vi "_Dequeue CSMQ.vi"(8 "Error in":errorcluster caption="Error in (no error)", 9 "Dequeue Timeout(0ms)":i32, 10 "State(s) in (\"\")":string, 11 "CSMQ in":T1) -> (0 "Error out":errorcluster, 2 "States Out":string, 3 "CSMQ out":T1)   [LabVIEW 2014, in "Communicable State Machine.lvlib"]
uses:
  Communicable State Machine.lvlib
  _CSMObj.ctl
  Priority Queue/Priority Queue.lvclass
  Typedef/_CSM_MODE.ctl
  _CSMObj-Data.ctl
  Typedef/_CSM Status Change Event Data.ctl
  Priority Queue/Priority Queue.lvclass/Priority Queue.ctl
  AdvanceAPI/CSM - Message Type.ctl
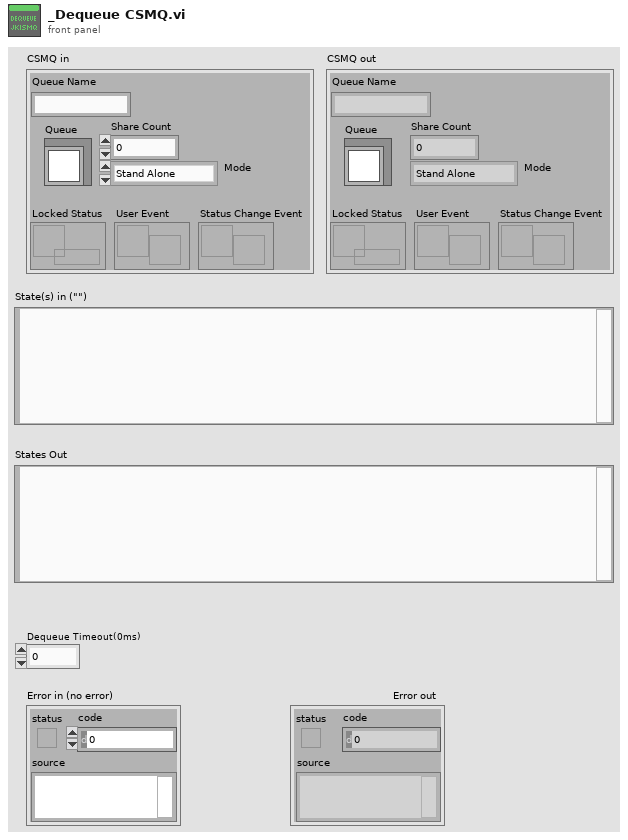
[diagram p1: front panel]
types:
  T1 = typedef "Communicable State Machine.lvlib/_CSMObj.ctl" = cluster{"Queue Name":string, "Mode":T2, "Share Count":i32, "Queue":refnum<class "Priority Queue.lvclass">, "Locked Status":refnum<data-value>, "User Event":refnum<user-event>, "Status Change Event":refnum<user-event>}
  T2 = typedef "Communicable State Machine.lvlib/_CSM_MODE.ctl" = enum16{"Stand Alone", "CSM", "Action Worker"}
  T3 = typedef "Communicable State Machine.lvlib/CSM - Message Type.ctl" = enum16{"Async", "Async without Reply", "Sync"}
  T4 = typedef "_CSMObj-Data.ctl" = cluster{"Locked?":bool, "RemoteMessge?":bool}
  T5 = typedef "Communicable State Machine.lvlib/_Cross CSM State Data.ctl" = cluster{"Msg Type":T6, "state":string, "args":string, "source":string, "RespQ":refnum<queue>, "Response For Message":T7, "Target":string}
  T6 = typedef "Communicable State Machine.lvlib/_CSM_MSG_TYPE.ctl" = enum16{"Sync Message(-@)", "Async Message(->)", "Async without Response(->|)", "Async Response", "Broadcast(-><status>)", "Broadcast(-><interrupt>)", "Request to Post Message", "Request to Post Message without Reply", "Request to Publish Status"}
  T7 = typedef "Communicable State Machine.lvlib/_CSM_Response Source Message.ctl" = cluster{"State":string, "Arguments":string, "Error":errorcluster}
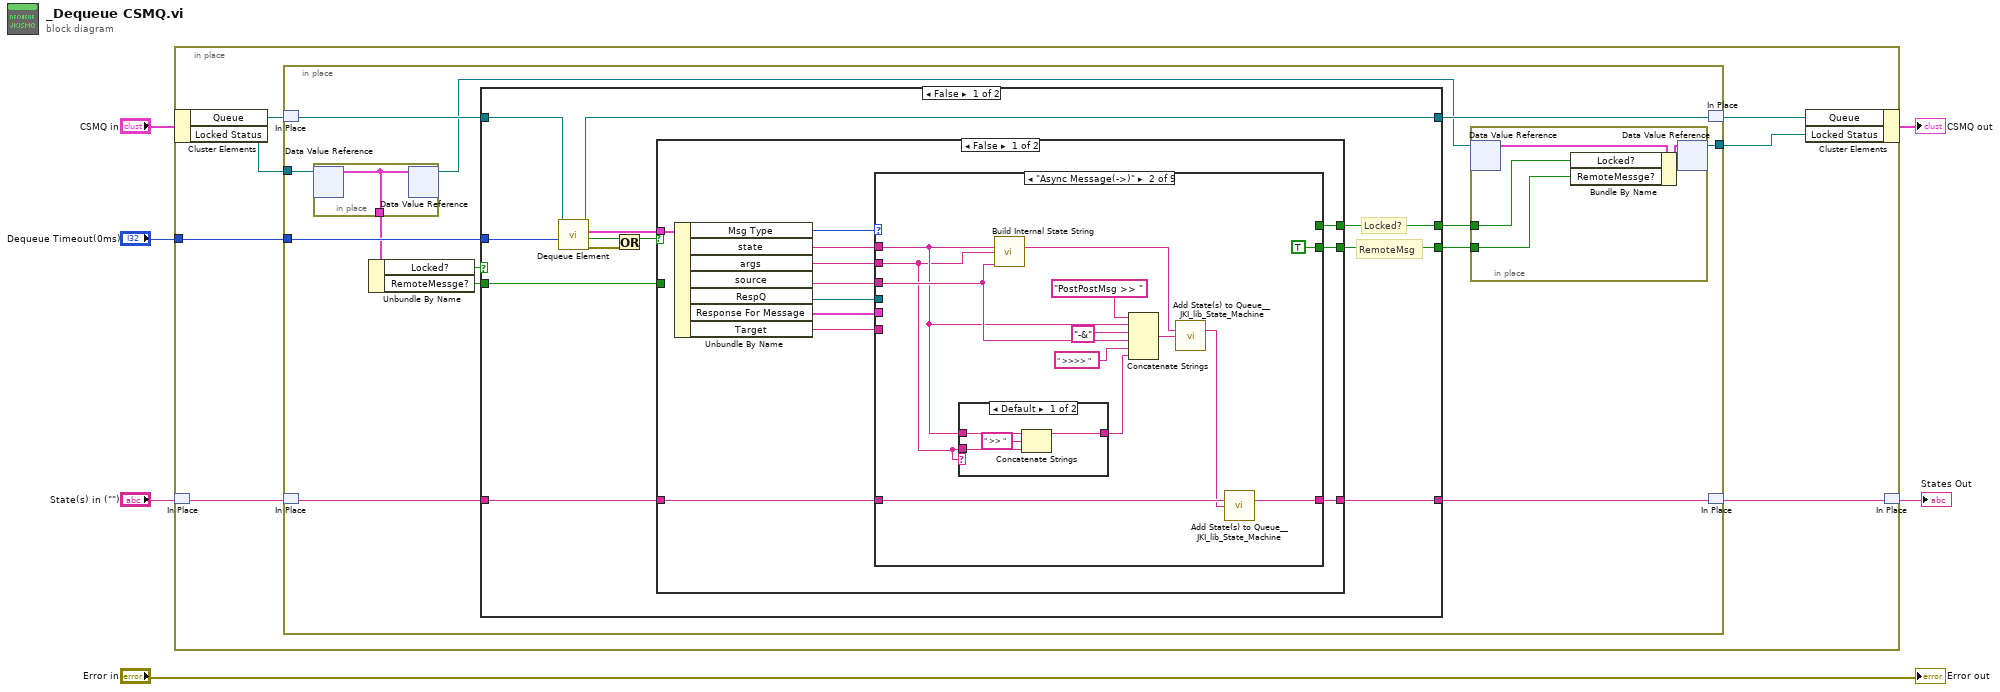
[diagram p0: block diagram]
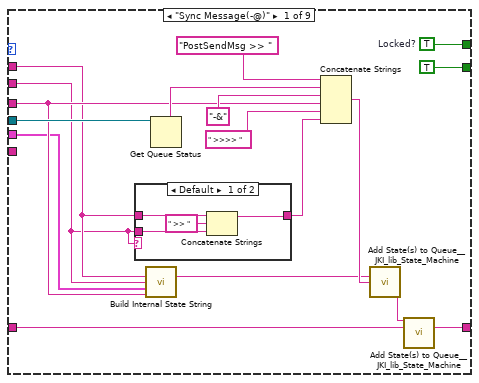
[diagram p2: hidden frame]
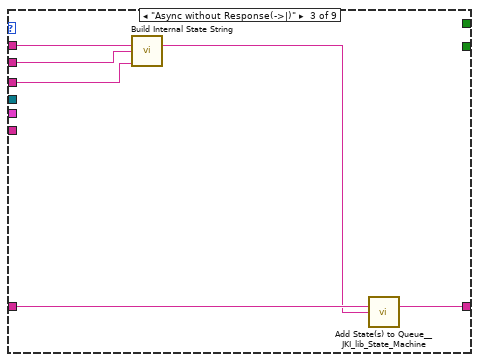
[diagram p5: hidden frame]
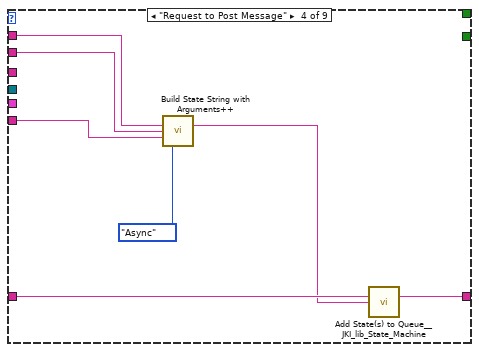
[diagram p6: hidden frame]
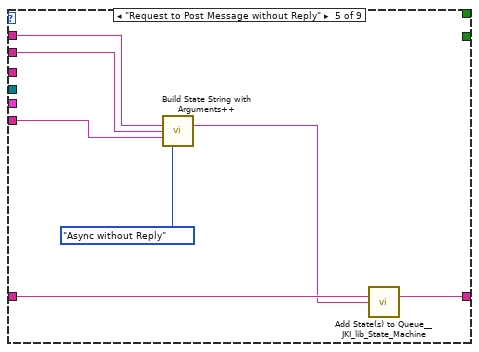
[diagram p7: hidden frame]
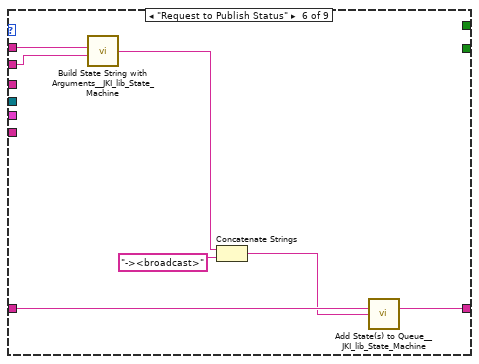
[diagram p8: hidden frame]
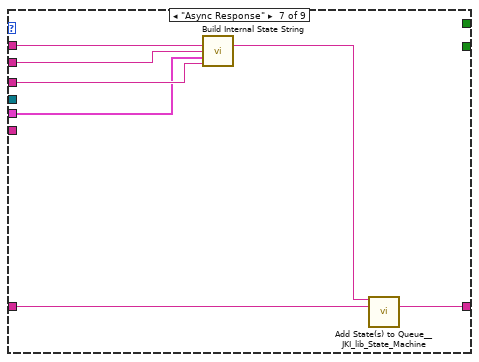
[diagram p9: hidden frame]
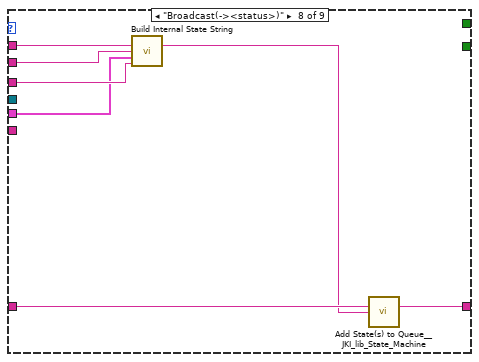
[diagram p10: hidden frame]
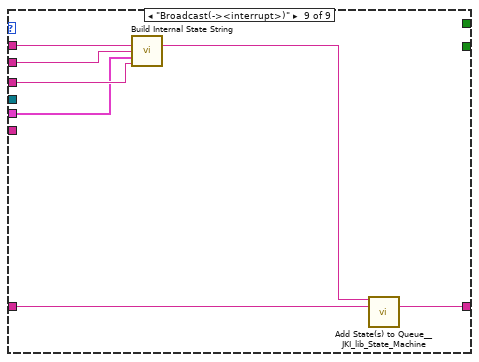
[diagram p11: hidden frame]
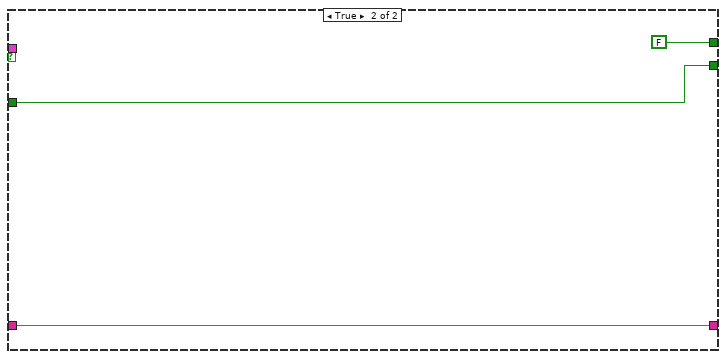
[diagram p12: hidden frame]
diagram:
  n1 = in-place "In Place Element Structure" {
    in-place-border: "Dequeue Timeout(0ms)" -> [w11]
    n2 = in-place-cluster #1("CSMQ in") -> ("Queue"=w13:refnum<class "Priority Queue.lvclass">, "Locked Status"=w8:refnum<data-value>)
    n3 = in-place-match #2("State(s) in (\"\")") -> (w10:string)
    n4 = in-place {
      in-place-border: w11 -> [w24]
      in-place-border: w8 -> [w21]
      in-place-border: [w18] -> w7
      n5 = in-place-match #3(w13) -> (w25:refnum<class "Priority Queue.lvclass">)
      n6 = in-place-match #4(w10) -> (w23:string)
      n7 = in-place {
        in-place-border: [w31] -> w20
        n8 = in-place-dvr #5(w21) -> (w31:T4)  [unwired: 1 out]
        n9 = in-place-dvr #5(w31) -> (w19:refnum<data-value>)  [unwired: 1 out]
      }
      n10 = Unbundle By Name(w20) -> ("Locked?"=w16:bool, "RemoteMessge?"=w14:bool)
      n11 = case shown="False" w16 {
        selector: w16 -> [_ w148]
        tunnel: [w42 w150] -> w26
        tunnel: w25 -> [w43 w150]
        tunnel: w24 -> [w41 _]
        tunnel: w23 -> [w39 w149]
        tunnel: [w38 w149] -> w22
        tunnel: [w37 w148] -> w17
        tunnel: [w33 w147] -> w15
        tunnel: w14 -> [w32 w147]
        frame False {
          # "RemoteMsg"
          # "Locked?"
          n12 = call "Dequeue Element.vi"("timeout in ms (-1)"=w41, "Priority Queue"=w43) -> ("error out"=w34:errorcluster, "timed out?"=w35:bool, "Cross JKI State Machine State"=w40:T5, "Priority Queue"=w42:refnum<class "Priority Queue.lvclass">)  [unwired: 5 in, 1 out]
          n13 = Or(x=w35, y=w34) -> (x .or. y?=w36:bool)
          n14 = case shown="False" w36 {
            tunnel: w39 -> [w55 w146]
            tunnel: [w54 w146] -> w38
            tunnel: w40 -> [w49 _]
            tunnel: [w48 FALSE] -> w37
            tunnel: [w44 w144] -> w33
            tunnel: w32 -> [_ w144]
            frame False {
              n15 = Unbundle By Name(w49) -> ("Msg Type"=w46:T6, "state"=w52:string, "args"=w51:string, "source"=w50:string, "RespQ"=w53:refnum<queue>, "Response For Message"=w47:T7, "Target"=w45:string)
              n16 = case shown="\"Async Message(->)\"" w46 {
                tunnel: w55 -> [w72 w90 w101 w108 w115 w122 w129 w136 w143]
                tunnel: [w71 w89 w100 w107 w114 w121 w128 w135 w142] -> w54
                tunnel: w53 -> [w70 _ _ _ _ _ _ _ _]
                tunnel: w52 -> [w57 w79 w97 w106 w113 w118 w125 w132 w139]
                tunnel: w51 -> [w56 w78 w99 w105 w112 w117 w127 w134 w141]
                tunnel: w50 -> [w61 w88 w98 _ _ _ w126 w133 w140]
                tunnel: [w63 _ _ _ _ _ _ _ _] -> w48
                tunnel: w47 -> [w58 _ _ _ _ _ w123 w131 w138]
                tunnel: w45 -> [_ _ _ w104 w111 _ _ _ _]
                tunnel: [TRUE TRUE _ _ _ _ _ _ _] -> w44
                frame "Sync Message(-@)" {
                  w63 = TRUE  # Locked?
                  n17 = case "Is arguments empty? If so, then do not append arguments" shown="Default" w56 {
                    tunnel: [w73 w77] -> w60
                    tunnel: w57 -> [w76 w77]
                    tunnel: w56 -> [w74 _]
                    frame Default {
                      n18 = Concatenate Strings(w76, " >> " ("string"), w74) -> (w73:string)
                    }
                    frame "" {
                    }
                  }
                  n19 = call "Build Internal State String.vi"("State"=w57, "Arguments (\"\")"=w56, ">> Response Source Message >>"=w58, "Source (\"\")"=w61) -> ("State with Arguments"=w66:string)  [unwired: 11 in]
                  n20 = Get Queue Status(queue=w70) -> (queue name=w65:string)  [unwired: 2 in, 7 out]
                  n21 = Concatenate Strings("PostSendMsg >> " ("State(s) at Back (\"\")"), w65, "-&" ("string"), w61, " >>>> " ("string"), w60) -> (w67:string)
                  n22 = call <vilib>:"Add State(s) to Queue__JKI_lib_State_Machine.vi"("State(s) in (\"\")"=w66, "State(s) at Back (\"\")"=w67) -> ("States Out"=w69:string)  [unwired: 13 in]
                  n23 = call <vilib>:"Add State(s) to Queue__JKI_lib_State_Machine.vi"("State(s) in Front (\"\")"=w69, "State(s) in (\"\")"=w72) -> ("States Out"=w71:string)  [unwired: 13 in]
                }
                frame "Async Message(->)" {
                  n24 = case "Is arguments empty? If so, then do not append arguments" shown="Default" w78 {
                    tunnel: [w91 w95] -> w81
                    tunnel: w79 -> [w94 w95]
                    tunnel: w78 -> [w92 _]
                    frame Default {
                      n25 = Concatenate Strings(w94, " >> " ("string"), w92) -> (w91:string)
                    }
                    frame "" {
                    }
                  }
                  n26 = call "Build Internal State String.vi"("State"=w79, "Arguments (\"\")"=w78, "Source (\"\")"=w88) -> ("State with Arguments"=w84:string)  [unwired: 12 in]
                  n27 = Concatenate Strings("PostPostMsg >> " ("State(s) at Back (\"\")"), w79, "-&" ("string"), w88, " >>>> " ("string"), w81) -> (w83:string)
                  n28 = call <vilib>:"Add State(s) to Queue__JKI_lib_State_Machine.vi"("State(s) in (\"\")"=w84, "State(s) at Back (\"\")"=w83) -> ("States Out"=w87:string)  [unwired: 13 in]
                  n29 = call <vilib>:"Add State(s) to Queue__JKI_lib_State_Machine.vi"("State(s) in (\"\")"=w90, "State(s) at Back (\"\")"=w87) -> ("States Out"=w89:string)  [unwired: 13 in]
                }
                frame "Async without Response(->|)" {
                  n30 = call "Build Internal State String.vi"("State"=w97, "Arguments (\"\")"=w99, "Source (\"\")"=w98) -> ("State with Arguments"=w96:string)  [unwired: 12 in]
                  n31 = call <vilib>:"Add State(s) to Queue__JKI_lib_State_Machine.vi"("State(s) in (\"\")"=w101, "State(s) at Back (\"\")"=w96) -> ("States Out"=w100:string)  [unwired: 13 in]
                }
                frame "Request to Post Message" {
                  n32 = call "Build State String with Arguments++.vi"("State"=w106, "Arguments (\"\")"=w105, "Target Module (\"\")"=w104, "Type"=CSM_-_Message_Type."Async") -> ("State with Arguments"=w103:string)  [unwired: 11 in]
                  n33 = call <vilib>:"Add State(s) to Queue__JKI_lib_State_Machine.vi"("State(s) in (\"\")"=w108, "State(s) at Back (\"\")"=w103) -> ("States Out"=w107:string)  [unwired: 13 in]
                }
                frame "Request to Post Message without Reply" {
                  n34 = call "Build State String with Arguments++.vi"("State"=w113, "Arguments (\"\")"=w112, "Target Module (\"\")"=w111, "Type"=CSM_-_Message_Type."Async without Reply") -> ("State with Arguments"=w110:string)  [unwired: 11 in]
                  n35 = call <vilib>:"Add State(s) to Queue__JKI_lib_State_Machine.vi"("State(s) in (\"\")"=w115, "State(s) at Back (\"\")"=w110) -> ("States Out"=w114:string)  [unwired: 13 in]
                }
                frame "Request to Publish Status" {
                  n36 = call <vilib>:"Build State String with Arguments__JKI_lib_State_Machine.vi"("Arguments (\"\")"=w117, "State"=w118) -> ("State with Arguments"=w116:string)  [unwired: 4 in]
                  n37 = Concatenate Strings(w116, "-><broadcast>" ("string")) -> (w119:string)
                  n38 = call <vilib>:"Add State(s) to Queue__JKI_lib_State_Machine.vi"("State(s) in (\"\")"=w122, "State(s) at Back (\"\")"=w119) -> ("States Out"=w121:string)  [unwired: 13 in]
                }
                frame "Async Response" {
                  n39 = call "Build Internal State String.vi"("State"=w125, "Arguments (\"\")"=w127, ">> Response Source Message >>"=w123, "Source (\"\")"=w126) -> ("State with Arguments"=w124:string)  [unwired: 11 in]
                  n40 = call <vilib>:"Add State(s) to Queue__JKI_lib_State_Machine.vi"("State(s) in Front (\"\")"=w124, "State(s) in (\"\")"=w129) -> ("States Out"=w128:string)  [unwired: 13 in]
                }
                frame "Broadcast(-><status>)" {
                  n41 = call "Build Internal State String.vi"("State"=w132, "Arguments (\"\")"=w134, ">> Response Source Message >>"=w131, "Source (\"\")"=w133) -> ("State with Arguments"=w130:string)  [unwired: 11 in]
                  n42 = call <vilib>:"Add State(s) to Queue__JKI_lib_State_Machine.vi"("State(s) in (\"\")"=w136, "State(s) at Back (\"\")"=w130) -> ("States Out"=w135:string)  [unwired: 13 in]
                }
                frame "Broadcast(-><interrupt>)" {
                  n43 = call "Build Internal State String.vi"("State"=w139, "Arguments (\"\")"=w141, ">> Response Source Message >>"=w138, "Source (\"\")"=w140) -> ("State with Arguments"=w137:string)  [unwired: 11 in]
                  n44 = call <vilib>:"Add State(s) to Queue__JKI_lib_State_Machine.vi"("State(s) in Front (\"\")"=w137, "State(s) in (\"\")"=w143) -> ("States Out"=w142:string)  [unwired: 13 in]
                }
              }
            }
            frame True {
            }
          }
        }
        frame True {
        }
      }
      n45 = in-place {
        in-place-border: w17 -> [w28]
        in-place-border: w15 -> [w27]
        n46 = in-place-dvr #6(w19) -> (w30:T4)  [unwired: 1 out]
        n47 = Bundle By Name(cluster=w30, "Locked?"=w28, "RemoteMessge?"=w27) -> (w29:T4)
        n48 = in-place-dvr #6(w29) -> (w18:refnum<data-value>)  [unwired: 1 out]
      }
      n49 = in-place-match #3(w26) -> (w12:refnum<class "Priority Queue.lvclass">)
      n50 = in-place-match #4(w22) -> (w9:string)
    }
    n51 = in-place-cluster #1("Queue"=w12, "Locked Status"=w7) -> (→"CSMQ out":T1)
    n52 = in-place-match #2(w9) -> (→"States Out":string)
  }
  "Error out" <- "Error in"
